vi "Keyence.Main.Scan.vi"(4 "ReadImg":bool, 5 "Retries":i32, 6 "Timeout_ms":i32, 7 "Bank":u8, 8 "error in (no error)":errorcluster, 9 "IP":string, 10 "ImgPath":path, 11 "TCP Network Connection in":refnum<k5>) -> (0 "error out":errorcluster, 1 "Code":T1, 2 "File name":path, 3 "TCP Network Connection out":refnum<k5>)   [LabVIEW 2016]
uses:
  LowLevel/Keyence.CodeDetails.ctl
  LowLevel/Keyence.Global.vi
  Station/Station.Global.vi
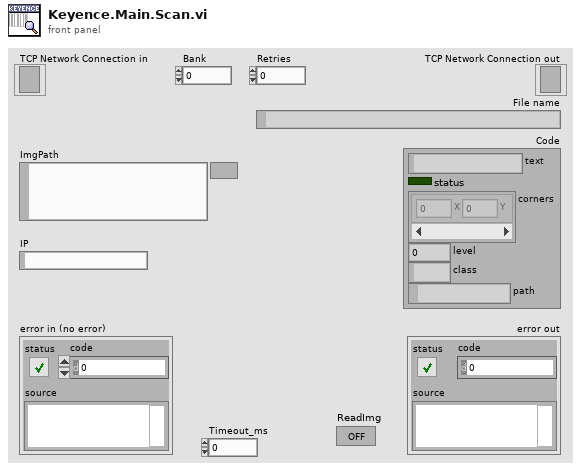
[diagram p1: front panel]
types:
  T1 = typedef "Keyence.CodeDetails.ctl" = cluster{"text":string, "status":bool, "corners":cluster{"X":i32, "Y":i32}[], "level":u8, "class":string, "path":path}
  T2 = typedef "NI_FTP.lvlib/FTP Session.ctl" = refnum<k5>
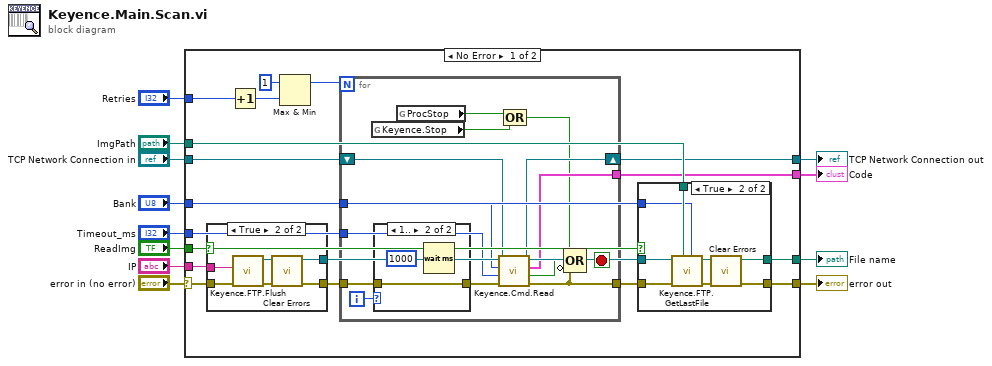
[diagram p0: block diagram]
diagram:
  n1 = case shown="No Error" "error in (no error)" {
    selector: "error in (no error)" -> [w13 w63]
    tunnel: [w30 _] -> w12
    tunnel: "Bank" -> [w28 _]
    tunnel: "ReadImg" -> [w27 _]
    tunnel: "IP" -> [w26 _]
    tunnel: "ImgPath" -> [w25 _]
    tunnel: [w23 _] -> w7
    tunnel: [w22 w63] -> w6
    tunnel: "Timeout_ms" -> [w19 _]
    tunnel: "Retries" -> [w16 _]
    tunnel: [w15 w62] -> w3
    tunnel: "TCP Network Connection in" -> [w14 w62]
    frame No Error {
      n2 = case shown="True" w27 {
        tunnel: w13 -> [w31 w34]
        tunnel: [w31 w36] -> w24
        tunnel: w26 -> [_ w35]
        tunnel: [_ w32] -> w29
        frame False {
        }
        frame True {
          n3 = call "Keyence.FTP.Flush.vi"("error in (no error)"=w34, "host"=w35) -> ("error out"=w33:errorcluster, "FTP Session out"=w32:T2)  [unwired: 8 in]
          n4 = call <vilib>:"Clear Errors.vi"("error in (no error)"=w33) -> ("error out"=w36:errorcluster)  [unwired: 5 in, 1 out]
        }
      }
      n5 = Increment(x=w16) -> (x+1=w17:i32)
      n6 = Max & Min(x=1, y=w17) -> (max(x,y)=w20:i32)  [unwired: 1 out]
      n7 = for {
        N: w20 -> [_]
        shift-right: [w49] -> w15
        shift-left: w14 -> [w50]
        tunnel: w24 -> [w43]
        tunnel: [w44] -> w21
        tunnel: w28 -> [w48]
        tunnel: w19 -> [w47]
        tunnel: [w40] -> w23
        i -> [w41]
        stop <- w45 stop-if-true
        n8 = global read "Keyence.Global.vi" "Keyence.Stop"() -> (w38:bool)
        n9 = case shown="1.." w41 {
          tunnel: [w51 w53] -> w42
          tunnel: w43 -> [w51 w53]
          frame Default {
          }
          frame 1.. {
            n10 = Wait (ms)(milliseconds to wait=u32 1000) -> ()  [unwired: 1 out]
          }
        }
        n11 = global read "Station.Global.vi" "ProcStop"() -> (w39:bool)
        n12 = call "Keyence.Cmd.Read.vi"("error in (no error)"=w42, "Timeout [ms] (1000)"=w47, "Bank"=w48, "connection ID"=w50) -> ("error out"=w44:errorcluster, "read ok"=w46:bool, "Code"=w40:T1, "connection ID out"=w49:refnum<k5>)  [unwired: 4 in]
        n13 = Compound Arithmetic op=OR(w39, w38) -> (w37:bool)
        n14 = Compound Arithmetic op=OR(w37, w46, invert w44) -> (w45:bool)
      }
      n15 = case shown="True" w27 {
        tunnel: w21 -> [w54 w59]
        tunnel: [w54 w60] -> w22
        tunnel: [_ w61] -> w30
        tunnel: w25 -> [_ w58]
        tunnel: w28 -> [_ w56]
        tunnel: w29 -> [_ w55]
        frame False {
        }
        frame True {
          n16 = call "Keyence.FTP.GetLastFile.vi"("Bank (0)"=w56, "LogPath"=w58, "error in (no error)"=w59, "FTP Session out"=w55) -> ("error out"=w57:errorcluster, "File name"=w61:path)  [unwired: 6 in]
          n17 = call <vilib>:"Clear Errors.vi"("error in (no error)"=w57) -> ("error out"=w60:errorcluster)  [unwired: 5 in, 1 out]
        }
      }
    }
    frame Error {
    }
  }
  "File name" <- w12
  "Code" <- w7
  "error out" <- w6
  "TCP Network Connection out" <- w3
